vi "FineContrast_cleaned inputs.vi"(0 "LFA in":refnum<class "LightField Automation.lvclass">, 1 "PZC in":string="GPIB/0:4,0", 2 "Photodiode in":refnum<visa-resource-name>, 3 "ESP 301 COM":refnum<visa-resource-name>="COM1", 4 "LFA error in":errorcluster, 5 "PZC error in":errorcluster, 6 "Photodiode error in":errorcluster {"code" format="%.0x"}, 7 "ESP 301 error in":errorcluster, 8 "Scan Translation Exp Params":T2, 9 "PZC Pos (usteps)":refnum<vi>, 10 "Scan Translation Params":T3, 11 "Pause button":refnum<vi>, 12 "Contrast Oscillations":refnum<vi>, 13 "Stop button":refnum<vi>, 14 "Contrast 1D Spectrum":refnum<vi>, 15 "Progess Bar":refnum<vi>, 16 "Shutter Device":refnum<vi>, 18 "Shutter":refnum<vi>) -> (17 "PZAPos & InstPow":dbl[][](array[numeric]), 19 "Spectra vs PZA":i32[][](array[numeric]), 20 "LFA out":refnum<class "LightField Automation.lvclass">, 21 "PZC out":string, 22 "Photodiode out":refnum<visa-resource-name>, 23 "ESP 301 COM out":refnum<visa-resource-name>="COM1", 24 "LFA error out":errorcluster, 25 "PZC error out":errorcluster, 26 "Photodiode error out":errorcluster {"code" format="%.0x"}, 27 "ESP 301 error out":errorcluster)   [LabVIEW 2019]
uses:
  D:/Users/manip-thz/Documents/Controle_Manip_2020/Thorlabs.MotionControl.KCube.SolenoidCLI.dll
  Thorlabs.MotionControl.KCube.SolenoidCLI.dll
  Light Field/lightfield-automation-labview/LightField Automation.lvclass
  TypeDefs/AcqMode.ctl
panel:
  out "KCube Shutter On?":bool
  out "range":dbl
  out "LinT End pos (mm)":dbl
  out "LinT Step Pos (mm)":dbl
  out "LinT Start Pos (mm)":dbl
  out "Scan Contrast Ctrls":refnum<vi>[](array[refnum])
  out "InstPow":dbl[](array[numeric])
  out "ExcPow_uW":dbl
  in  "ExcWL_nm":dbl
  out "WavelengthCalibration":dbl[](array[numeric])
  out "x+y":dbl
  out "PZA Positions":i32[](array[numeric])
  out "Contrast values":i32[](array[numeric])
  out "Contrast 1D Spectrum":cluster{dbl[], dbl[]}(graph) caption="64.0°"
  out "Contrast Oscillations":cluster{dbl[], dbl[]}(graph)
  in  "Acq Mode":T1=enum."Spectrum" caption="Mode :"
  in  "Acq Time (ms) 2":dbl=500.0 caption="Acq Time :" min=0.0 max=360000.0 step=50.0
  in  "Pause Contrast":bool
  in  "Stop Contrast":bool
  out "PZC Position Readout (usteps)":dbl caption="Readout (usteps)" min=-8.0 max=392.0
  out "Scan Spectrum Progess Bar":u8(slide) scale=0.0..100.0
  out "KCube Shutter Device Reference":refnum<k24>
  out "Shutter Ctrls":u16(ring)
  in  "CCD ROI":T4(ring)
  in  "Accumulations":dbl=1.0
  in  "LinTFine Step":dbl
  in  "LinTFine End":dbl
  in  "LinTFine Start":dbl
  # "ms"
types:
  T1 = typedef "AcqMode.ctl" = enum16{"Image", "Spectrum", "APD 1", "APD 2", "APD 1+2"}
  T2 = cluster{"Exposure Time (ms)":dbl, "Accumulations":dbl, "Excitation Wavelength (nm)":dbl, "Acq Mode":T1, "CCD ROI":enum16{"Custom ROI", "Full sensor", "Binned full sensor"}, "KCube Shutter On?":bool}
  T3 = cluster{"LinT Start Pos (mm)":dbl, "LinT Step Pos (mm)":dbl, "LinT End pos (mm)":dbl, "LinTFine Start Pos (usteps)":dbl, "LinTFines Step Pos (usteps)":dbl, "LinTFine End Pos (usteps)":dbl}
  T4 = enum16{"Custom ROI", "Full sensor", "Binned full sensor"}
  T5 = enum16{"Contrast", "Spectre", "Polarisation", "Time Trace", "XY Intensity Map"}
  T6 = enum16{"Image", "Spectrum", "APD 1", "APD 2", "APD 1+2"}
  T7 = cluster{"Image":dbl[][][], "Frame Size":cluster{"F":i32, "Y":i32, "X":i32}}[]
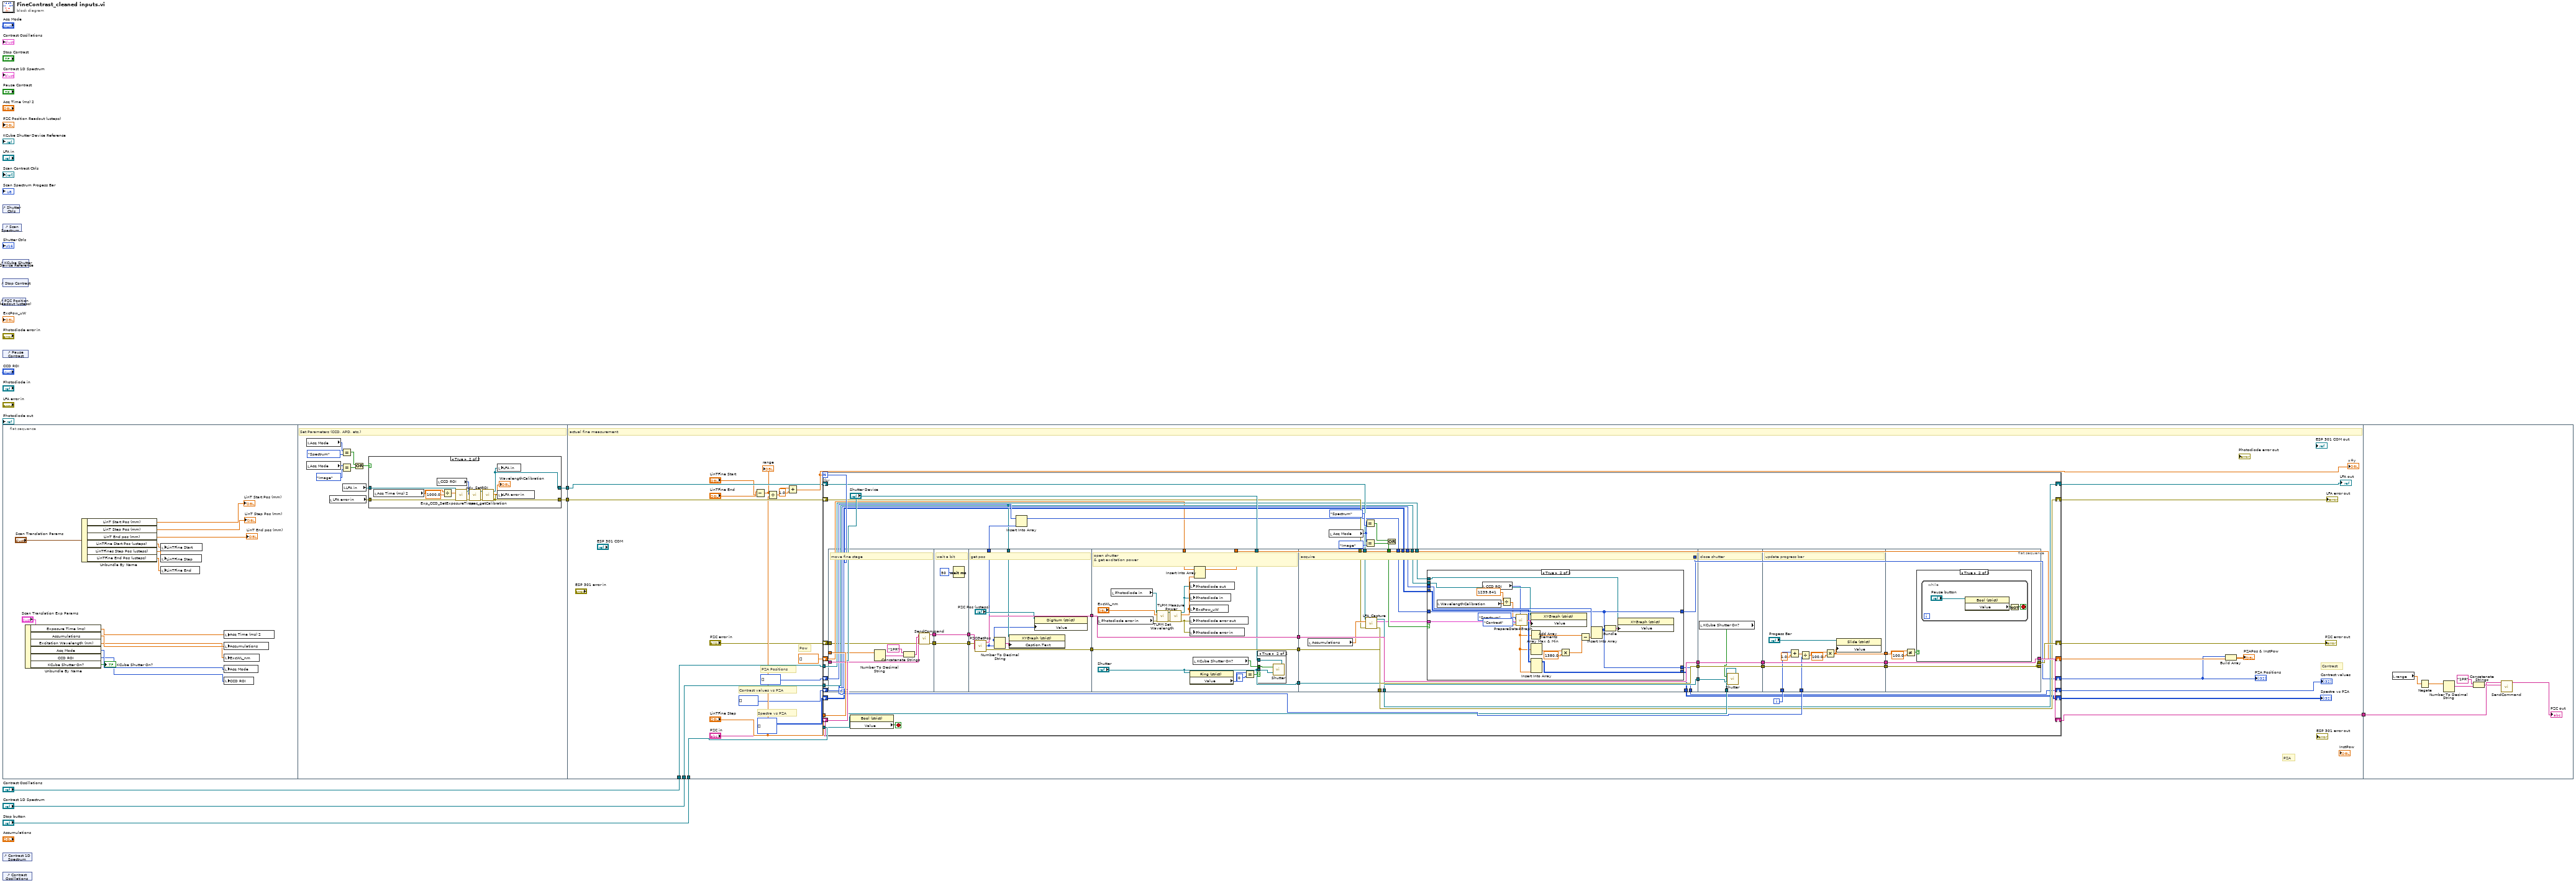
[diagram p0: block diagram]
diagram:
  n1 = control-ref of="Shutter Ctrls"() -> ()  [unwired: 1 out]
  n2 = control-ref of="Scan Spectrum Progess Bar"() -> ()  [unwired: 1 out]
  n3 = control-ref of="KCube Shutter Device Reference"() -> ()  [unwired: 1 out]
  n4 = control-ref of="Stop Contrast"() -> ()  [unwired: 1 out]
  n5 = control-ref of="PZC Position Readout (usteps)"() -> ()  [unwired: 1 out]
  n6 = control-ref of="Pause Contrast"() -> ()  [unwired: 1 out]
  n7 = flat-sequence {
    tunnel: [w24] -> w6
    tunnel: [w23] -> w5
    tunnel: w6 -> [w71]
    tunnel: w5 -> [w70]
    tunnel: "Stop button" -> [w66]
    tunnel: "Contrast 1D Spectrum" -> [w65]
    tunnel: "Contrast Oscillations" -> [w64]
    tunnel: [w47] -> w1
    tunnel: w1 -> [w230]
    frame #0 {
      n8 = Unbundle By Name("Scan Translation Exp Params") -> ("Exposure Time (ms)"=w12:dbl, "Accumulations"=w11:dbl, "Excitation Wavelength (nm)"=w10:dbl, "Acq Mode"=w9:T1, "CCD ROI"=w8:T4, "KCube Shutter On?"=→"KCube Shutter On?":bool)
      n9 = Unbundle By Name("Scan Translation Params") -> ("LinT Start Pos (mm)"=→"LinT Start Pos (mm)":dbl, "LinT Step Pos (mm)"=→"LinT Step Pos (mm)":dbl, "LinT End pos (mm)"=→"LinT End pos (mm)":dbl, "LinTFine Start Pos (usteps)"=w18:dbl, "LinTFines Step Pos (usteps)"=w19:dbl, "LinTFine End Pos (usteps)"=w20:dbl)
      n10 = local write "LinTFine Start"(w18) -> ()
      n11 = local write "LinTFine Step"(w19) -> ()
      n12 = local write "LinTFine End"(w20) -> ()
      n13 = local write "Acq Time (ms) 2"(w12) -> ()
      n14 = local write "Accumulations"(w11) -> ()
      n15 = local write "ExcWL_nm"(w10) -> ()
      n16 = local write "Acq Mode"(w9) -> ()
      n17 = local write "CCD ROI"(w8) -> ()
    }
    frame #1 {
      # "Set Parameters (CCD, APD, etc.)"
      n18 = local read "Acq Mode"() -> (w31:T1)
      n19 = local read "Acq Mode"() -> (w27:T1)
      n20 = local read "LFA error in"() -> (w22:errorcluster)
      n21 = Equal?(x=w31, y=AcqMode."Spectrum" ("Acq Mode")) -> (x = y?=w29:bool)
      n22 = Equal?(x=w27, y=AcqMode."Image" ("Acq Mode")) -> (x = y?=w26:bool)
      n23 = local read "LFA in"() -> (w21:refnum<class "LightField Automation.lvclass">)
      n24 = Or(x=w29, y=w26) -> (x .or. y?=w25:bool)
      n25 = case shown="True" w25 {
        tunnel: [w33 w40] -> w24
        tunnel: [w32 w39] -> w23
        tunnel: w22 -> [w32 w44]
        tunnel: w21 -> [w33 w43]
        frame False {
        }
        frame True {
          n26 = local read "Acq Time (ms) 2"() -> (w37:dbl)
          n27 = local read "CCD ROI"() -> (w34:T4)
          n28 = Divide(x=w37, y=1000.0) -> (x/y=w35:dbl)
          n29 = call "Exp_CCD_SetExposureTime.vi"("error in (no error)"=w44, "Exposure Time (s)"=w35, "LightField Automation in"=w43) -> ("error out"=w45:errorcluster, "LightField Automation out"=w46:refnum<class "LightField Automation.lvclass">)  [unwired: 7 in]
          n30 = call "Adv_SetROI.vi"("error in (no error)"=w45, "ROI"=w34, "LightField Automation in"=w46) -> ("error out"=w41:errorcluster, "LightField Automation out"=w42:refnum<class "LightField Automation.lvclass">)  [unwired: 7 in]
          n31 = call "spec_getCalibration.vi"("error in (no error)"=w41, "LightField Automation in"=w42) -> ("error out"=w39:errorcluster, "ColumnCalibration"=→"WavelengthCalibration":dbl[], "LightField Automation out"=w40:refnum<class "LightField Automation.lvclass">)  [unwired: 7 in]
          n32 = local write "LFA in"(w40) -> ()
          n33 = local write "LFA error in"(w39) -> ()
        }
      }
    }
    frame #2 {
      # "PZA Positions"
      # "Pow"
      # "Spectra vs PZA"
      # "Contrast values vs PZA"
      # "Contrast"
      # "PZA"
      # "actual fine measurement"
      n34 = Subtract(x="LinTFine End", y="LinTFine Start") -> (x-y=w57:dbl)
      "range" <- w57
      n35 = Divide(x=w57, y="LinTFine Step") -> (x/y=w56:dbl)
      n36 = Add(x=w56, y=1.0) -> (x+y=w73:dbl)
      "x+y" <- w73
      n37 = for {
        N: w73 -> [w106]
        tunnel: "LinTFine Step" -> [w122]
        shift-right: [w101] -> w47
        shift-left: "PZC in" -> [w120]
        shift-right: [w100] -> w72
        shift-left: "PZC error in" -> [w121]
        shift-right: [w89] -> w69
        shift-left: w71 -> [w91]
        shift-right: [w88] -> w68
        shift-left: w70 -> [w90]
        shift-right: [w78] -> w60
        shift-left: i32[] [] -> [w86]
        shift-right: [w77] -> w67
        shift-left: i32[] [] -> [w83]
        tunnel: w66 -> [w85]
        tunnel: w65 -> [w81]
        tunnel: w64 -> [w80]
        shift-right: [w76] -> w63
        shift-left: i32[][] [] -> [w79]
        shift-right: [w74] -> w62
        shift-left: dbl[] [] -> [w75]
        i -> [w107]
        stop <- w102 stop-if-true
        n38 = flat-sequence {
          tunnel: w122 -> [w130]
          tunnel: [w126] -> w119
          tunnel: [w125] -> w117
          tunnel: w121 -> [w124]
          tunnel: w120 -> [w123]
          tunnel: w119 -> [w133]
          tunnel: [w133] -> w118
          tunnel: w117 -> [w132]
          tunnel: [w132] -> w116
          tunnel: w118 -> [w141]
          tunnel: w116 -> [w140]
          tunnel: [w139] -> w115
          tunnel: [w138] -> w114
          tunnel: [w134] -> w87
          tunnel: w81 -> [w136]
          tunnel: w115 -> [w159]
          tunnel: w114 -> [w158]
          tunnel: "Shutter Device" -> [w154]
          tunnel: [w159] -> w113
          tunnel: [w158] -> w112
          tunnel: ["Shutter"] -> w98
          tunnel: w75 -> [w147]
          tunnel: [w145] -> w74
          tunnel: w113 -> [w180]
          tunnel: w112 -> [w179]
          tunnel: [w180] -> w111
          tunnel: [w179] -> w110
          tunnel: [w177] -> w99
          tunnel: w98 -> [w177]
          tunnel: w91 -> [w176]
          tunnel: w90 -> [w175]
          tunnel: [w174] -> w89
          tunnel: [w173] -> w88
          tunnel: w84 -> [w172]
          tunnel: w83 -> [w170]
          tunnel: w82 -> [w169]
          tunnel: w81 -> [w168]
          tunnel: w80 -> [w167]
          tunnel: w79 -> [w166]
          tunnel: [w165] -> w78
          tunnel: [w164] -> w77
          tunnel: [w163] -> w76
          tunnel: w111 -> [w210]
          tunnel: w110 -> [w209]
          tunnel: [w210] -> w109
          tunnel: [w209] -> w108
          tunnel: w99 -> [w208]
          tunnel: "Shutter Device" -> [w207]
          tunnel: w109 -> [w220]
          tunnel: w108 -> [w219]
          tunnel: w107 -> [w213]
          tunnel: w106 -> [w212]
          tunnel: [w220] -> w105
          tunnel: [w219] -> w104
          tunnel: [w211] -> w103
          tunnel: [w221] -> _
          tunnel: [w225] -> w101
          tunnel: w105 -> [w225]
          tunnel: w104 -> [w221]
          tunnel: w103 -> [w223]
          tunnel: [w221] -> w100
          frame #0 {
            # "move fine stage"
            n39 = Number To Decimal String(number=w130) -> (decimal integer string=w128:string)  [unwired: 1 in]
            n40 = Concatenate Strings("1PR", w128) -> (w127:string)
            n41 = call "SendCommand.vi"("error in"=w124, "Command"=w127, "Instrument Channel"=w123) -> ("error out"=w125:errorcluster, "Instrument Channel out"=w126:string)  [unwired: 7 in]
          }
          frame #1 {
            # "wait a bit"
            n42 = Wait (ms)(milliseconds to wait=u32 50) -> ()  [unwired: 1 out]
          }
          frame #2 {
            # "get pos"
            n43 = call "PZCGetPos.vi"("error in"=w140, "Instrument Channel"=w141) -> ("Instrument Channel Out"=w139:string, "Position"=w134:i32, "error out"=w138:errorcluster)
            n44 = Number To Decimal String(number=w134) -> (decimal integer string=w135:string)  [unwired: 1 in]
            n45 = property class="XYGraph (strict)"(reference=w136, "Caption.Text"=w135) -> ()  [unwired: 1 in, 2 out]
            n46 = property class="DigNum (strict)"(reference="PZC Pos (usteps)", "Value"=w134) -> ()  [unwired: 1 in, 2 out]
          }
          frame #3 {
            # "open shutter\n& get excitation power"
            n47 = local read "Photodiode error in"() -> (w150:errorcluster)
            n48 = local read "Photodiode in"() -> (w149:refnum<visa-resource-name>)
            n49 = call <instrlib>:"TLPM Set Wavelength.vi"("error in (no error)"=w150, "Wavelength (0.0)"="ExcWL_nm", "instrument handle"=w149) -> ("error out"=w151:errorcluster, "instrument handle out"=w152:refnum<visa-resource-name>)  [unwired: 7 in]
            n50 = call <instrlib>:"TLPM Measure Power.vi"("error in (no error)"=w151, "instrument handle"=w152) -> ("error out"=w143:errorcluster, "Power"=w146:dbl, "instrument handle out"=w144:refnum<visa-resource-name>)  [unwired: 7 in]
            n51 = local write "Photodiode out"(w144) -> ()
            n52 = local write "Photodiode in"(w144) -> ()
            n53 = local write "ExcPow_uW"(w146) -> ()
            n54 = local write "Photodiode error out"(w143) -> ()
            n55 = local write "Photodiode error in"(w143) -> ()
            n56 = property class="Ring (strict)"(reference="Shutter") -> ("Value"=w155:u16)  [unwired: 1 in, 2 out]
            n57 = local read "KCube Shutter On?"() -> (w142:bool)
            n58 = Insert Into Array(array=w147, new element=w146) -> (w145:dbl[])  [unwired: 1 in]
            n59 = Equal?(x=w155, y=u16 0) -> (x = y?=w156:bool)
            n60 = case shown="True" w156 {
              tunnel: "Shutter" -> [_ w162]
              tunnel: w154 -> [_ w161]
              tunnel: w142 -> [_ w160]
              frame False {
              }
              frame True {
                n61 = call "Shutter.vi"("KCube Shutter Device Reference 2"=w161, "Shutter Ctrls 2"=w162, "Shutter on?"=w160) -> ()
              }
            }
          }
          frame #4 {
            # "acquire"
            n62 = local read "Accumulations"() -> (w178:dbl)
            n63 = call "LFA_Capture.vi"("error in (no error)"=w175, "Frames"=w178, "LightField Automation in"=w176) -> ("error out"=w173:errorcluster, "Data"=w171:T7, "LightField Automation out"=w174:refnum<class "LightField Automation.lvclass">)  [unwired: 6 in]
            n64 = case shown="True" w172 {
              tunnel: w171 -> [_ w205]
              tunnel: w170 -> [w182 w204]
              tunnel: w169 -> [w183 w202]
              tunnel: [w183 w202] -> w165
              tunnel: [w182 w201] -> w164
              tunnel: w168 -> [_ w200]
              tunnel: w167 -> [_ w199]
              tunnel: w166 -> [w181 w196]
              tunnel: [w181 w195] -> w163
              frame False {
              }
              frame True {
                n65 = local read "WavelengthCalibration"() -> (w188:dbl[])
                n66 = local read "CCD ROI"() -> (w184:T4)
                n67 = Divide(x=1239.841, y=w188) -> (x/y=w186:dbl[])
                n68 = call "PrepareData4Graph.vi"("Wavelength nm"=w186, "DataLF"=w205, "CCD ROI"=w184, "AcqMode"=T6."Spectrum", "Data type"=T5."Contrast") -> ("Spectrum"=w197:cluster{"Array 2":dbl[], "Array":dbl[]}, "PLInt out"=w191:dbl[])  [unwired: 2 in, 2 out]
                n69 = Add Array Elements(numeric array=w191) -> (sum=w194:dbl)
                n70 = property class="XYGraph (strict)"(reference=w200, "Value"=w197) -> ()  [unwired: 1 in, 2 out]
                n71 = Array Max & Min(array=w191) -> (min value=w190:dbl)  [unwired: 3 out]
                n72 = Insert Into Array(array=w196, new element=w191) -> (w195:i32[][])  [unwired: 2 in]
                n73 = Multiply(x=w190, y=1380.0) -> (x*y=w189:dbl)
                n74 = Subtract(x=w194, y=w189) -> (x-y=w193:dbl)
                n75 = Insert Into Array(array=w204, new element=w193) -> (w201:i32[])  [unwired: 1 in]
                n76 = Bundle(w202, w201) -> (w203:cluster{i32[], i32[]})  [unwired: 1 in]
                n77 = property class="XYGraph (strict)"(reference=w199, "Value"=w203) -> ()  [unwired: 1 in, 2 out]
              }
            }
          }
          frame #5 {
            # "close shutter"
            n78 = local read "KCube Shutter On?"() -> (w206:bool)
            n79 = call "Shutter.vi"("KCube Shutter Device Reference 2"=w207, "Shutter Ctrls 2"=w208, "Shutter on?"=w206) -> ()
          }
          frame #6 {
            # "update progress bar"
            n80 = Add(x=w213, y=1.0) -> (x+y=w217:dbl)
            n81 = Divide(x=w217, y=w212) -> (x/y=w216:dbl)
            n82 = Multiply(x=w216, y=100.0) -> (x*y=w211:dbl)
            n83 = property class="Slide (strict)"(reference="Progess Bar", "Value"=w211) -> ()  [unwired: 1 in, 2 out]
          }
          frame #7 {
            n84 = Not Equal?(x=w223, y=100.0) -> (x != y?=w222:bool)
            n85 = case shown="True" w222 {
              frame False {
              }
              frame True {
                n86 = while {
                  stop <- w227 stop-if-true
                  n87 = property class="Bool (strict)"(reference="Pause button") -> ("Value"=w228:bool)  [unwired: 1 in, 2 out]
                  n88 = Not(x=w228) -> (.not. x?=w227:bool)
                }
              }
            }
          }
        }
        n89 = property class="Bool (strict)"(reference=w85) -> ("Value"=w102:bool)  [unwired: 1 in, 2 out]
        n90 = Insert Into Array(array=w86, new element=w87) -> (w82:i32[])  [unwired: 1 in]
        n91 = local read "Acq Mode"() -> (w96:T1)
        n92 = Equal?(x=w96, y=AcqMode."Spectrum" ("Acq Mode")) -> (x = y?=w92:bool)
        n93 = Equal?(x=w96, y=AcqMode."Image" ("Acq Mode")) -> (x = y?=w93:bool)
        n94 = Or(x=w92, y=w93) -> (x .or. y?=w84:bool)
      }
      "LFA out" <- w69
      "LFA error out" <- w68
      "Contrast values" <- w67
      "PZC error out" <- w72
      "Spectra vs PZA" <- w63
      "PZA Positions" <- w60
      n95 = Build Array(w60, w62) -> (→"PZAPos & InstPow":dbl[][])
    }
    frame #3 {
      n96 = local read "range"() -> (w233:dbl)
      n97 = Negate(x=w233) -> (-x=w232:dbl)
      n98 = Number To Decimal String(number=w232) -> (decimal integer string=w235:string)  [unwired: 1 in]
      n99 = Concatenate Strings("1PR", w235) -> (w234:string)
      n100 = call "SendCommand.vi"("Command"=w234, "Instrument Channel"=w230) -> ("Instrument Channel out"=→"PZC out":string)  [unwired: 8 in, 1 out]
    }
  }
  n101 = control-ref of="Contrast 1D Spectrum"() -> ()  [unwired: 1 out]
  n102 = control-ref of="Contrast Oscillations"() -> ()  [unwired: 1 out]
